vi "FSD.vi"() -> ()   [LabVIEW 2019]
uses:
  <vilib>/imath/engines/lvmath2/RunTimeEngine/RangeToken/NIMS_Range.vi
  <instcachedir>/0/NIMS_Range_0856D726B6B24596B614846B21C682A9.lvgen/NIMS_Range_0856D726B6B24596B614846B21C682A9_000.vi
  <vilib>/imathl/engines/lvmath/Functions/Error Handling/Create Error.vi
  <vilib>/imath/engines/lvmath2/RunTimeEngine/BuiltInFunctions/sawtooth/NIMS_sawtooth(RV, rs).vi
  <vilib>/imath/engines/lvmath2/RunTimeEngine/ErrorHandling/NIMS_Error From Error Code.vi
  <vilib>/imath/engines/lvmath2/RunTimeEngine/BuiltInFunctions/square/NIMS_square.vi
  <instcachedir>/0/NIMS_square_8BE126634BDB49EE87F69273AACFE816.lvgen/NIMS_square_8BE126634BDB49EE87F69273AACFE816_001.vi
  <vilib>/imath/engines/lvmath2/RunTimeEngine/BuiltInFunctions/zeros/NIMS_V=zeros(I32,I32).vi
  <vilib>/imath/engines/lvmath2/RunTimeEngine/ErrorHandling/NIMS_Create Error From Enums.vi
  <vilib>/imath/engines/lvmath2/RunTimeEngine/VariableToken/NIMS_VariableToken_CondDefined.vi
  <instcachedir>/0/NIMS_VariableToken_CondDefined_FCC6C4723AB84F8A81236997BED5B96C.lvgen/NIMS_VariableToken_CondDefined_FCC6C4723AB84F8A81236997BED5B96C_003.vi
  <vilib>/imath/engines/lvmath2/RunTimeEngine/BuiltInFunctions/repeatmx/NIMS_repeatmx(GM, I32, I32).vi
  <instcachedir>/0/NIMS_repeatmx(GM, I32, I32)_9340A36EE73A4C0A822BF3A4FC82B863.lvgen/NIMS_repeatmx(GM, I32, I32)_9340A36EE73A4C0A822BF3A4FC82B863_000.vi
  <vilib>/imath/engines/lvmath2/RunTimeEngine/BuiltInFunctions/length/NIMS_length(GV).vi
  <instcachedir>/0/NIMS_length(GV)_08A3D13377FD4E4B96F5795FBF3698FA.lvgen/NIMS_length(GV)_08A3D13377FD4E4B96F5795FBF3698FA_000.vi
  <vilib>/imath/engines/lvmath2/RunTimeEngine/BuiltInFunctions/mean/NIMS_RS=mean(RV,I32).vi
  <instcachedir>/0/NIMS_Range_0856D726B6B24596B614846B21C682A9.lvgen/NIMS_Range_0856D726B6B24596B614846B21C682A9_001.vi
  <vilib>/imath/engines/lvmath2/RunTimeEngine/RangeToken/NIMS_Range_R2 - Float.vi
  <instcachedir>/0/NIMS_Range_R2 - Float_34C0770B58484855BEFB6CBFA9AC9324.lvgen/NIMS_Range_R2 - Float_34C0770B58484855BEFB6CBFA9AC9324_000.vi
  <vilib>/imath/engines/lvmath2/RunTimeEngine/CommandStatement/MC_CommandStatement_break.vi
  <vilib>/imath/engines/lvmath2/RunTimeSupport/NIMS_Error if Not Equal.vi
  <instcachedir>/0/NIMS_Error if Not Equal_559A38B1E9844760937E85B04C5ADA21.lvgen/NIMS_Error if Not Equal_559A38B1E9844760937E85B04C5ADA21_000.vi
  <vilib>/imath/engines/lvmath2/RunTimeEngine/ArithmeticOperatorToken/NIMS_ArithmeticOperator_times.vi
  <instcachedir>/0/NIMS_ArithmeticOperator_times_BC2A7BF92F8245379E8C6B3F6BDCD4B7.lvgen/NIMS_ArithmeticOperator_times_BC2A7BF92F8245379E8C6B3F6BDCD4B7_000.vi
  <vilib>/imath/engines/lvmath2/RunTimeEngine/BuiltInFunctions/sum/NIMS_sum(GV).vi
  <instcachedir>/0/NIMS_sum(GV)_67F5EC36BC034E54A6BEC5B0673C00E5.lvgen/NIMS_sum(GV)_67F5EC36BC034E54A6BEC5B0673C00E5_000.vi
  <vilib>/imath/engines/lvmath2/RunTimeEngine/IndexReplace/NIMS V(S)=S.vi
  <instcachedir>/0/NIMS V(S)=S_B9932668475A4AEEB58CEEAB74E1195A.lvgen/NIMS V(S)=S_B9932668475A4AEEB58CEEAB74E1195A_000.vi
  <vilib>/imath/engines/lvmath2/RunTimeEngine/BuiltInFunctions/length/NIMS_length(GM).vi
  <instcachedir>/0/NIMS_length(GM)_47CEC356FCE0482D9BA47DC61C99F2C7.lvgen/NIMS_length(GM)_47CEC356FCE0482D9BA47DC61C99F2C7_000.vi
  <vilib>/imath/engines/lvmath2/RunTimeEngine/BuiltInFunctions/ones/NIMS_V=ones(I32,I32).vi
  <vilib>/imath/engines/lvmath2/RunTimeEngine/IndexRead/NIMS V(S).vi
  <instcachedir>/0/NIMS V(S)_0488751826AF41519A22953C041130DC.lvgen/NIMS V(S)_0488751826AF41519A22953C041130DC_000.vi
  <vilib>/imath/engines/lvmath2/RunTimeEngine/ArithmeticOperatorToken/NIMS_ArithmeticOperator_plus.vi
  <instcachedir>/0/NIMS_ArithmeticOperator_plus_A857F7369B7D4E138264023AAAB8243E.lvgen/NIMS_ArithmeticOperator_plus_A857F7369B7D4E138264023AAAB8243E_004.vi
  <vilib>/imath/engines/lvmath2/RunTimeEngine/NodeEndStatement/NIMS_NodeEndStatement_Get Vector.vi
  <instcachedir>/0/NIMS_NodeEndStatement_Get Vector_5FE5044D2CCC4FE7BE3AE4771B6280C5.lvgen/NIMS_NodeEndStatement_Get Vector_5FE5044D2CCC4FE7BE3AE4771B6280C5_001.vi
  <vilib>/imath/engines/lvmath/Functions/Error Handling/MergeErrorsWrapper.vi
  <vilib>/imath/engines/lvmath2/RunTimeEngine/NodeEndStatement/NIMS_NodeEndStatement_Output.vi
  <instcachedir>/0/NIMS_NodeEndStatement_Output_53EC0D466D134D7ABD903AC30B43404B.lvgen/NIMS_NodeEndStatement_Output_53EC0D466D134D7ABD903AC30B43404B_001.vi
  <instcachedir>/0/NIMS_NodeEndStatement_Output_53EC0D466D134D7ABD903AC30B43404B.lvgen/NIMS_NodeEndStatement_Output_53EC0D466D134D7ABD903AC30B43404B_005.vi
  <vilib>/imath/engines/lvmath2/RunTimeEngine/ErrorHandling/NIMS_Finalize Error.vi
  <vilib>/Utility/file.llb/Write Delimited Spreadsheet (DBL).vi
panel:
  in  "Save to .txt":bool
  in  "wave .txt file":path
  in  "?":T1(tab)
  out "Input Signal":waveform(dbl)(graph)
  out "an":dbl[](graph)
  out "bn":dbl[](graph)
  out "a0":dbl
  out "an":dbl[](array[numeric])
  out "bn":dbl[](array[numeric])
  out "Reconstructed Signal":waveform(dbl)(graph)
  in  "Waveform":T2(ring)
  in  "Number of \nFourier coeffs (N)":dbl
  in  "Period":dbl
  in  "Amplitude":dbl
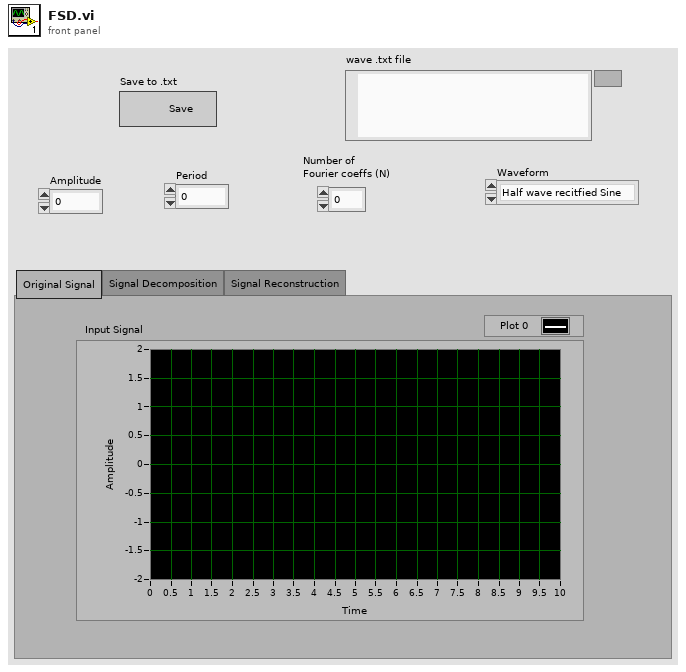
[diagram p1: front panel]
types:
  T1 = enum32{"Original Signal", "Signal Decomposition", "Signal Reconstruction"}
  T2 = enum16{"Half wave recitfied Sine ", "Square", "Sawtooth", "Triangular"}
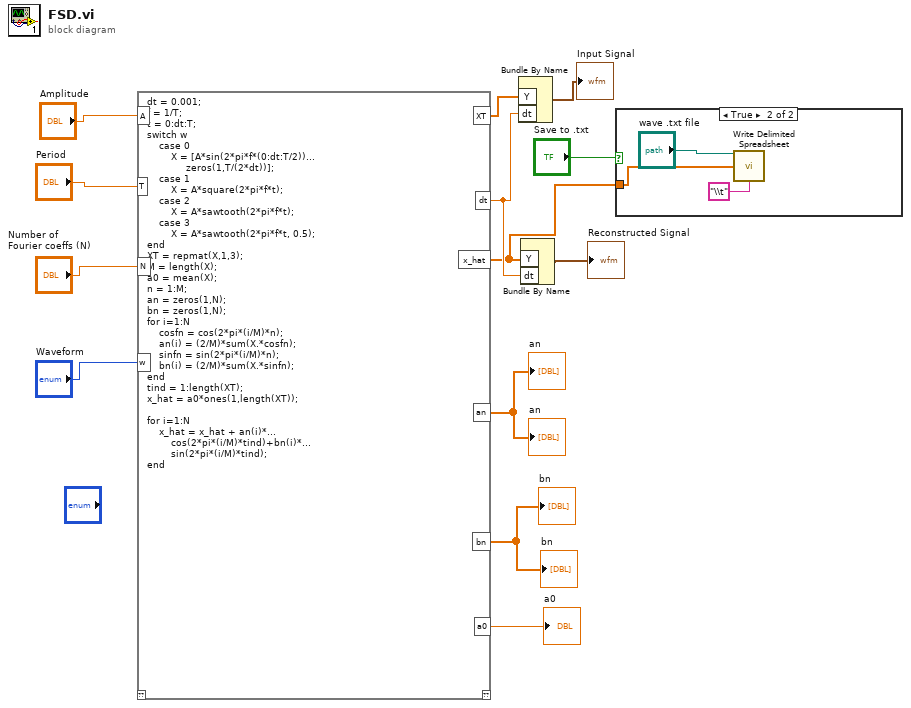
[diagram p0: block diagram]
diagram:
  n1 = mathscript code="dt = 0.001; \nf = 1/T;\nt = 0:dt:T;\nswitch w\n    case 0\n        X = [A*sin(2*pi*f*(0:dt:T/2))...\n             zeros(1,T/(2*dt))];\n    case 1\n        X = A*square(2*pi*f*t);\n    case 2\n        X = A*sawtooth(2*pi*f*t);\n    case 3\n        X = A*sawtooth(2*pi*f*t, 0.5);\nend\nXT = repmat(X,1,3);\nM = length(X);\na0 = mean(X);\nn = 1:M;\nan = zeros(1,N);\nbn = zeros(1,N);\nfor i=1:N\n    cosfn = cos(2*pi*(i/M)*n);\n    an(i) = (2/M)*sum(X.*cosfn);\n    sinfn = sin(2*pi*(i/M)*n);\n    bn(i) = (2/M)*sum(X.*sinfn);\nend\ntind = 1:length(XT);\nx_hat = a0*ones(1,length(XT));\n\nfor i=1:N\n    x_hat = x_hat + an(i)*...\n        cos(2*pi*(i/M)*tind)+bn(i)*...\n        sin(2*pi*(i/M)*tind);\nend"("A"="Amplitude", "T"="Period", "N"="Number of \nFourier coeffs (N)", "w"="Waveform") -> ("XT"=w9:dbl[], "dt"=w5:dbl, "x_hat"=w2:dbl[], "an"=→"an" →"an":dbl[], "bn"=→"bn" →"bn":dbl[], "a0"=→"a0":dbl)  [unwired: 1 in, 1 out]
  n2 = Bundle By Name("Y"=w9, "dt"=w5) -> (→"Input Signal":waveform(dbl))  [unwired: 1 in]
  n3 = Bundle By Name("Y"=w2, "dt"=w5) -> (→"Reconstructed Signal":waveform(dbl))  [unwired: 1 in]
  n4 = case shown="True" "Save to .txt" {
    tunnel: w2 -> [_ w15]
    frame False {
    }
    frame True {
      n5 = call-poly <vilib>:"Write Delimited Spreadsheet.vi"("file path (dialog if empty)"="wave .txt file", "1D data"=w15, "delimiter (\\t)"="\\t" ("delimiter (\\t)")) -> ()  [unwired: 11 in, 2 out]
    }
  }
